vi "Save Data in Locale.vi"(7 "Header":string[][](array[string]), 8 "error in (no error)":errorcluster, 9 "Channel":u16, 10 "Conditioned Data":dbl[][](array[numeric]), 11 "Father Of All Detectors in":refnum<class "Father Of All Detectors.lvclass">) -> (0 "error out":errorcluster, 2 "Conditioned Data Dup":dbl[][](array[numeric]), 3 "Father Of All Detectors out":refnum<class "Father Of All Detectors.lvclass">)   [LabVIEW 2026, in "TALOS.lvlib" / "Father Of All Detectors.lvlib" / "Father Of All Detectors.lvclass"]
uses:
  Father Of All Detectors.lvclass
  C:/LabVIEW Code/TALOS/talos/Classes/Hardware/Hardware.lvclass
  Ancestor/Ancestor/Ancestor.lvclass/Ancestor.ctl
  Support VIs/Circus Config Param - Core.vi
  <vilib>/AdvancedString/Delimited String to 1D String Array.vi
  <vilib>/AdvancedString/Delimited String to 1D String Array (string).vi
  Support VIs/Generate Error.vi
  Support VIs/Circus Root Path.vi
  Support VIs/TALOS Config Param.vi
  FGV/Error Memory/Get Error Description.vi
  Support VIs/Get PC name.vi
  Ancestor/Ancestor/Read ID.vi
  <vilib>/Utility/error.llb/Clear Errors.vi
  FGV/Error Memory/Error Memory Core.vi
  FGV/Error Memory/Error Crt Lvl checker.vi
  FGV/Error Memory/Error Memory Core.vi/40c8088d-b597-4017-91af-faa98e00292e.vi
  FGV/Error Memory/Error Memory Core.vi/d4a3ab98-063c-4e44-b43d-fbdcfe6c2be2.vi
  Support VIs/Global Memory.vi
  <vilib>/Utility/LVClass/Get LV Class Name.vi
  Support VIs/Is in Packed Library.vi
  Support VIs/TALOS Root path.vi
  Support VIs/Read CSV worksheet.vi
  Support VIs/Global Constants.vi
  <vilib>/Utility/error.llb/General Error Handler.vi
  <vilib>/Utility/config.llb/Open Config Data.vi
  <vilib>/Utility/config.llb/Get Section Names.vi
  <vilib>/Utility/config.llb/Get Key Names.vi
  <vilib>/Utility/config.llb/Read Key.vi
  <vilib>/Utility/config.llb/Read Key (String).vi
  <vilib>/Utility/config.llb/Close Config Data.vi
  <vilib>/Utility/error.llb/Search and Replace Pattern.vi
  <vilib>/Utility/error.llb/Search and Replace Pattern (string).vi
  <vilib>/Utility/file.llb/Write Delimited Spreadsheet (string).vi
  <vilib>/Utility/file.llb/Write Delimited Spreadsheet (DBL).vi
  Ancestor/Ancestor/Ancestor.lvclass
  <vilib>/Comparison/Equal/Equal Functor/Equal Functor.lvclass
  TALOS.lvlib
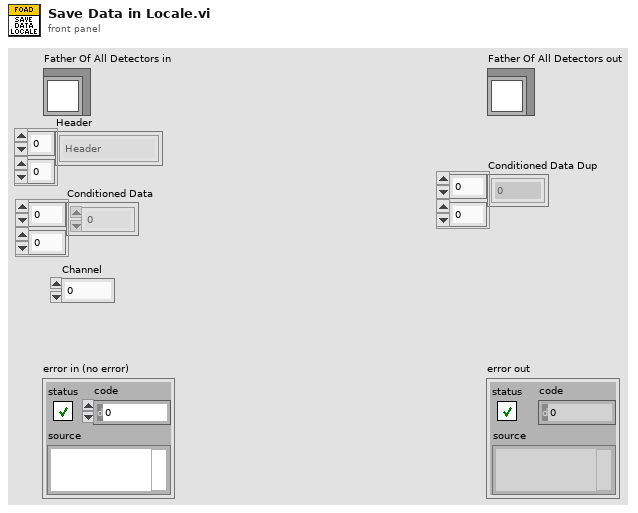
[diagram p1: front panel]
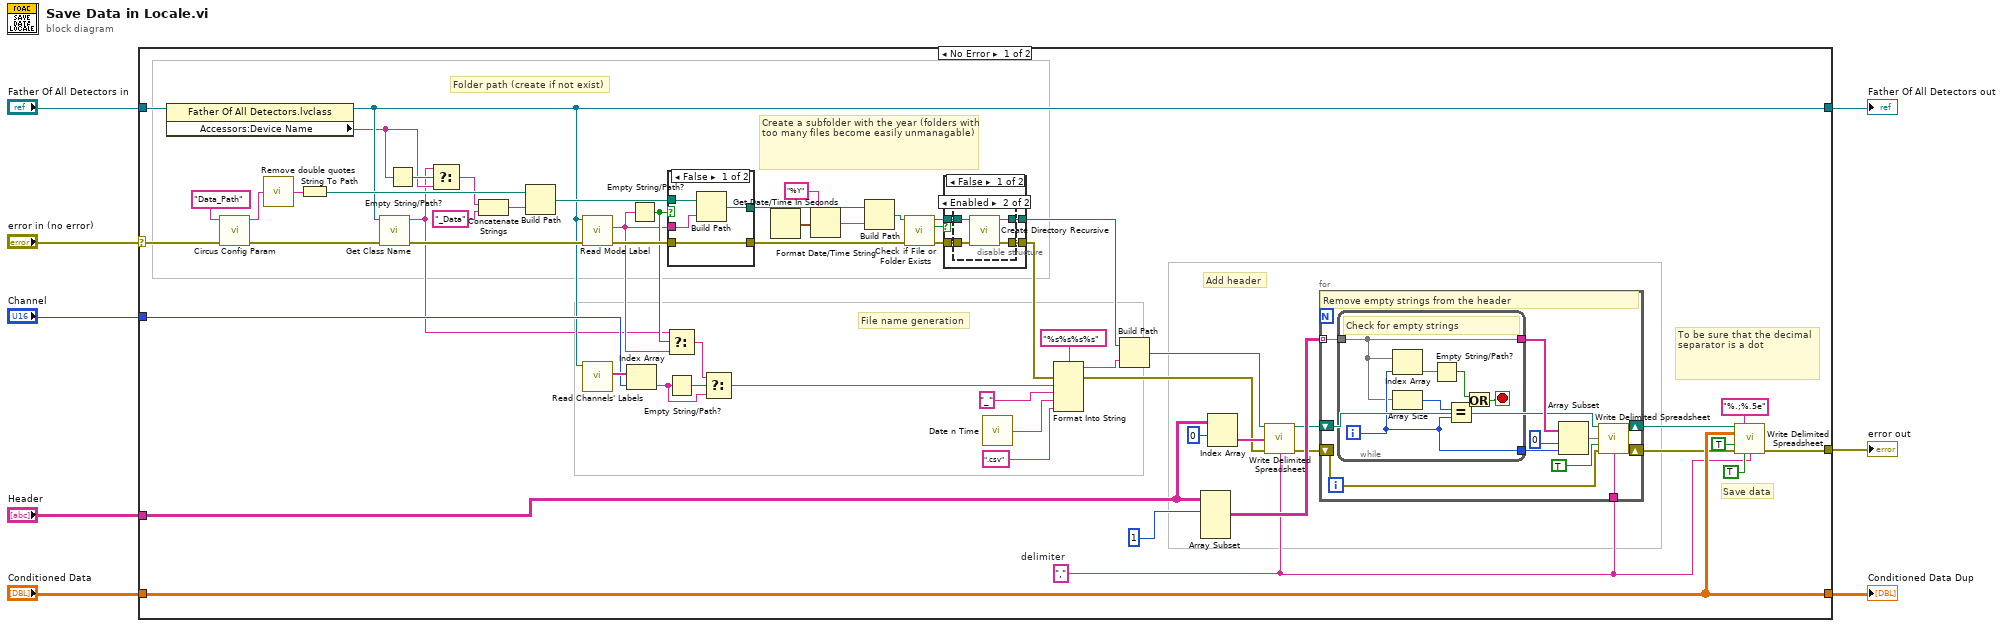
[diagram p0: block diagram]
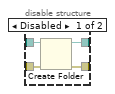
[diagram p2: hidden frame]
diagram:
  n1 = case shown="No Error" "error in (no error)" {
    selector: "error in (no error)" -> [w57 w106]
    tunnel: "Conditioned Data" -> [w34 w105]
    tunnel: "Channel" -> [w46 _]
    tunnel: "Father Of All Detectors in" -> [w20 w107]
    tunnel: [w19 w107] -> w4
    tunnel: [w62 w106] -> w5
    tunnel: [w34 w105] -> w6
    tunnel: "Header" -> [w30 _]
    frame No Error {
      w21 = ","  # delimiter
      # "Create a subfolder with the year (folders with too many files become easily unmanagable)"
      # "Add header"
      # "To be sure that the decimal separator is a dot"
      # "Save data"
      # "File name generation"
      # "Folder path (create if not exist)"
      n2 = property class="Father Of All Detectors.lvclass"(reference=w20) -> (reference out=w19:refnum<class "Father Of All Detectors.lvclass">, "Accessors:Device Name"=w16:string)  [unwired: 1 in, 1 out]
      n3 = call "Circus Config Param.vi"("error in (no error)"=w57, "Parameter Name"="Data_Path") -> ("error out"=w53:errorcluster, "Value"=w59:string)  [unwired: 8 in]
      n4 = call "Remove double quotes.vi"("Input string"=w59) -> ("Output string"=w56:string)  [unwired: 4 in]
      n5 = String To Path(string=w56) -> (path=w55:path)
      n6 = call "Get Class Name.vi"("error in (no error)"=w53, "object"=w19) -> ("error out"=w45:errorcluster, "Class Name"=w15:string)  [unwired: 8 in]
      n7 = Empty String/Path?(string/path=w16) -> (empty?=w17:bool)
      n8 = Select(t=w15, s=w17, f=w16) -> (s? t:f=w14:string)
      n9 = Concatenate Strings(w14, "_Data" ("string")) -> (w52:string)
      n10 = Build Path(base path=w55, name or relative path=w52) -> (appended path=w44:path)
      n11 = call-dynamic "Read Mode Label.vi"("error in (no error)"=w45, "Father Of All Detectors in"=w19) -> ("error out"=w43:errorcluster, "Mode Label"=w38:string)  [unwired: 7 in, 1 out]
      n12 = call-dynamic "Read Channels' Labels.vi"("Father Of All Detectors in"=w19) -> ("Channels' Labels"=w47:string[])  [unwired: 8 in, 2 out]
      n13 = Index Array(array=w47, index=w46) -> (element=w40:string)
      n14 = Empty String/Path?(string/path=w38) -> (empty?=w39:bool)
      n15 = Select(t=w15, s=w39, f=w38) -> (s? t:f=w37:string)
      n16 = Empty String/Path?(string/path=w40) -> (empty?=w41:bool)
      n17 = case shown="False" w39 {
        tunnel: w44 -> [w102 w104]
        tunnel: w43 -> [w99 w103]
        tunnel: [w101 w104] -> w13
        tunnel: [w99 w103] -> w42
        tunnel: w38 -> [w100 _]
        frame False {
          n18 = Build Path(base path=w102, name or relative path=w100) -> (appended path=w101:path)
        }
        frame True {
        }
      }
      n19 = Select(t=w37, s=w41, f=w40) -> (s? t:f=w36:string)
      n20 = Get Date/Time In Seconds() -> (seconds since 1Jan1904=w11:timestamp)
      n21 = Format Date/Time String(time format string (%c)="%Y", seconds (now)=w11) -> (date/time string=w9:string)  [unwired: 1 in]
      n22 = Build Path(base path=w13, name or relative path=w9) -> (appended path=w12:path)
      n23 = call <vilib>:"Check if File or Folder Exists.vi"("error in (no error)"=w42, "path"=w12) -> ("error out"=w50:errorcluster, "file or folder exists?"=w49:bool, "dup path"=w51:path)  [unwired: 7 in]
      n24 = case shown="False" w49 {
        tunnel: w51 -> [w88 w98]
        tunnel: w50 -> [w87 w97]
        tunnel: [w86 w98] -> w48
        tunnel: [w85 w97] -> w35
        frame False {
          n25 = disable-structure shown="Enabled" {
            disable-tunnel: w88 -> [w92 w96]
            disable-tunnel: w87 -> [w91 w95]
            disable-tunnel: [w90 w93] -> w86
            disable-tunnel: [w89 w94] -> w85
            frame Disabled {
              n26 = Create Folder(path (use dialog)=w92, error in=w91) -> (created path=w90:path, error out=w89:errorcluster)  [unwired: 1 in, 1 out]
            }
            frame Enabled {
              n27 = call <vilib>:"Create Directory Recursive.vi"("error in (no error)"=w95, "directory"=w96) -> ("error out"=w94:errorcluster, "directory copy"=w93:path)  [unwired: 3 in, 1 out]
            }
          }
        }
        frame True {
        }
      }
      n28 = call "Date n Time.vi"() -> ("Date & Time"=w61:string)  [unwired: 5 in]
      n29 = Format Into String(format string="%s%s%s%s", error in=w35, w36, "_", w61, ".csv" ("input 4")) -> (resulting string=w63:string, error out=w25:errorcluster)  [unwired: 1 in]
      n30 = Build Path(base path=w48, name or relative path=w63) -> (appended path=w27:path)
      n31 = Array Subset(array=w30, index (row)=1 ("index")) -> (w29:string[][])  [unwired: 3 in]
      n32 = Index Array(array=w30, index (row)=0) -> (element=w32:string[])  [unwired: 1 in]
      n33 = call-poly <vilib>:"Write Delimited Spreadsheet.vi"("file path (dialog if empty)"=w27, "1D data"=w32, "error in (no error)"=w25, "delimiter (\\t)"=w21) -> ("new file path (Not A Path if cancelled)"=w26:path, "error out"=w23:errorcluster)  [unwired: 10 in]
      n34 = for {
        tunnel: w29 -> [w75] mode=indexing
        tunnel: w21 -> [w71]
        shift-right: [w70] -> w24
        shift-left: w23 -> [w69]
        shift-right: [w68] -> w22
        shift-left: w26 -> [w72]
        # "Remove empty strings from the header"
        n35 = while {
          tunnel: [w80] -> w77
          tunnel: w75 -> [w78]
          tunnel: [w78] -> w74
          i -> [w80]
          stop <- w82 stop-if-true
          # "Check for empty strings"
          n36 = Index Array(array=w78, index=w80) -> (element=w79:string)
          n37 = Array Size(array=w78) -> (size(s)=w84:i32)
          n38 = Empty String/Path?(string/path=w79) -> (empty?=w81:bool)
          n39 = Equal?(x=w84, y=w80) -> (x = y?=w83:bool)
          n40 = Or(x=w81, y=w83) -> (x .or. y?=w82:bool)
        }
        n41 = Array Subset(array=w74, index=0, length=w77) -> (w73:string[])
        n42 = call-poly <vilib>:"Write Delimited Spreadsheet.vi"("file path (dialog if empty)"=w72, "1D data"=w73, "append to file? (new file:F)"=TRUE, "error in (no error)"=w69, "delimiter (\\t)"=w71) -> ("new file path (Not A Path if cancelled)"=w68:path, "error out"=w70:errorcluster)  [unwired: 9 in]
      }
      n43 = call-poly <vilib>:"Write Delimited Spreadsheet.vi"("file path (dialog if empty)"=w22, "format (%.3f)"="%.;%.5e", "2D data"=w34, "append to file? (new file:F)"=TRUE, "error in (no error)"=w24, "transpose? (no:F)"=TRUE, "delimiter (\\t)"=w21) -> ("error out"=w62:errorcluster)  [unwired: 7 in, 1 out]
    }
    frame Error {
    }
  }
  "error out" <- w5
  "Father Of All Detectors out" <- w4
  "Conditioned Data Dup" <- w6
